vi "PollList.Channels.vi"(8 "error in (no error)":errorcluster, 11 "Node Ptr":T1=18446744073709551615 format="%.0x") -> (0 "error out":errorcluster, 2 "Tags":string[](array[string]), 3 "Refs":T1[](array[typedef]) format="%.0x")   [LabVIEW 2013, in "OPC UA Client System Explorer.lvlib"]
uses:
  OPC UA Client System Explorer.lvlib
  <vilib>/NI Veristand/Custom Device API/Custom Device Item Ref.ctl
  Shared/Constants.vi
  <vilib>/NI Veristand/Custom Device API/Get Item Property (Dependent Node Pointer).vi
  <vilib>/NI Veristand/Custom Device API/Get Item Property (String).vi
  <vilib>/NI Veristand/Custom Device API/Custom Device API.lvlib
  Shared/OPC UA Client Shared.lvlib
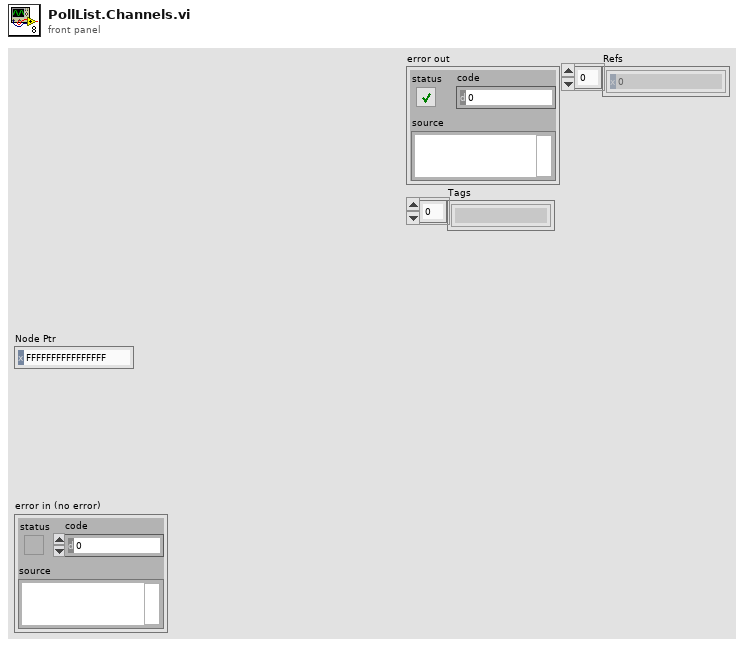
[diagram p1: front panel]
types:
  T1 = typedef "Custom Device API.lvlib/Custom Device Item Ref.ctl" = u64
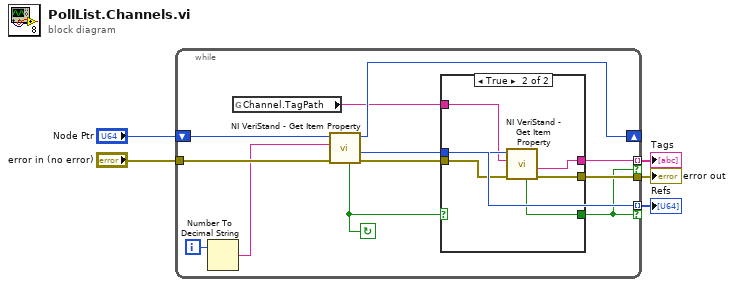
[diagram p0: block diagram]
diagram:
  n1 = while {
    tunnel: "error in (no error)" -> [w16]
    tunnel: [w11] -> w3
    tunnel: [w10] -> w1 mode=indexing if=w7
    shift-right: [w14] -> _
    shift-left: "Node Ptr" -> [w17]
    tunnel: [w9] -> w2 mode=indexing if=w7
    i -> [w15]
    stop <- w6 continue-if-true
    n2 = Number To Decimal String(number=w15) -> (decimal integer string=w13:string)  [unwired: 1 in]
    n3 = global read "Constants.vi" "Channel.TagPath"() -> (w8:string)
    n4 = call-poly <vilib>:"NI VeriStand - Get Item Property.vi"("error in (no error)"=w16, "Property Name"=w13, "Item Ref in"=w17) -> ("error out"=w12:errorcluster, "Dependent Node Ref"=w10:T1, "Item Ref out"=w14:T1, "Found"=w6:bool)  [unwired: 5 in]
    n5 = case shown="True" w6 {
      selector: w6 -> [w19 _]
      tunnel: w12 -> [w18 w25]
      tunnel: [w18 w24] -> w11
      tunnel: w10 -> [_ w23]
      tunnel: [_ w22] -> w9
      tunnel: w8 -> [_ w21]
      tunnel: [w19 w20] -> w7
      frame False {
      }
      frame True {
        n6 = call-poly <vilib>:"NI VeriStand - Get Item Property.vi"("error in (no error)"=w25, "Property Name"=w21, "Item Ref in"=w23) -> ("error out"=w24:errorcluster, "Value"=w22:string, "Found?"=w20:bool)  [unwired: 5 in, 1 out]
      }
    }
  }
  "error out" <- w3
  "Tags" <- w2
  "Refs" <- w1
